vi "Inject Attribute List.vi"(6 "Attributes Ref":refnum<data-value>, 8 "error in (no error)":errorcluster, 11 "Start Pre-Soak in":refnum<class "Set Desired Station.lvclass">) -> (0 "error out":errorcluster, 3 "Start Pre-Soak out":refnum<class "Set Desired Station.lvclass">)   [LabVIEW 2019, in "Set Desired Station.lvclass"]
uses:
  <vilib>/gpm_packages/@cs/Car-wash/Source/Process Steps/Set Desired Station/Set Desired Station.lvclass
  <vilib>/gpm_packages/@cs/lookup-table/Source/LookupTable/LookupTable.lvclass
  <vilib>/gpm_packages/@cs/lookup-table/Source/LookupTable/LookupTable.lvclass/LookupTable.ctl
  <vilib>/gpm_packages/@cs/Car-wash/Source/Process Steps/Set Desired Station/Set Desired Station.lvclass/Set Desired Station.ctl
  19c21afe-55da-448a-9dee-6152750ea2c7.vi
  <vilib>/gpm_packages/@cs/lookup-table/Source/LookupTable/Read Table Reference.vi
  19c21afe-55da-448a-9dee-6152750ea2c7.vi/19309c2b-5f09-4118-8446-a5db70bdcce7.vi
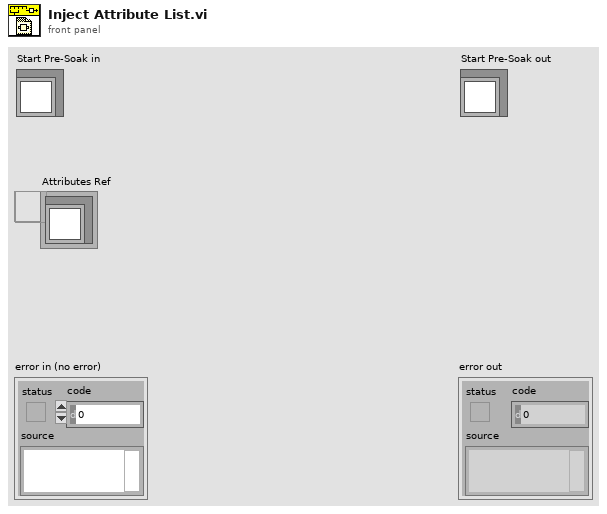
[diagram p1: front panel]
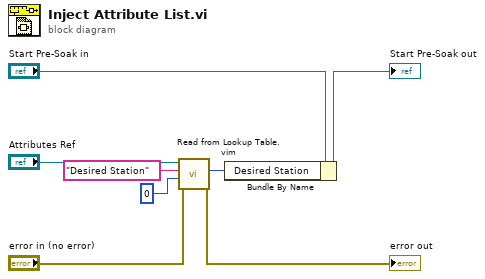
[diagram p0: block diagram]
diagram:
  n1 = call "Read from Lookup Table.vim"("error in (no error)"="error in (no error)", "Type"=u8 0, "Item Name"="Desired Station", "LookupTable Reference"="Attributes Ref") -> ("error out"=→"error out":errorcluster, "Value"=w6:u8)  [unwired: 4 in, 2 out]
  n2 = Bundle By Name(cluster="Start Pre-Soak in", "Desired Station"=w6) -> (→"Start Pre-Soak out":refnum<class "Set Desired Station.lvclass">)
